vi "UserEvent Driver.vi"(0 "Message":string, 5 "Data":variant, 11 "error in (no error)":errorcluster, 13 "Operations(Get Reference)":T1=enum."Get Reference") -> (4 "user event":refnum<user-event>, 15 "error out":errorcluster)   [LabVIEW 2014, in "Coding Platform.lvlib"]
uses:
  Coding Platform.lvlib
  Typedefs/User Event Data.ctl
  Typedefs/User Event Operations.ctl
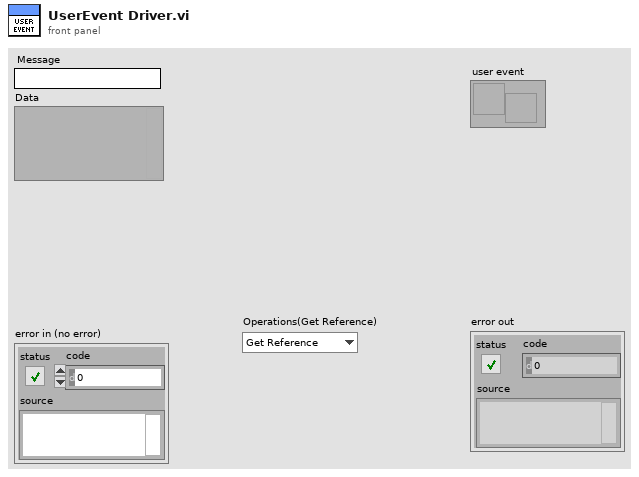
[diagram p1: front panel]
types:
  T1 = typedef "Coding Platform.lvlib/User Event Operations.ctl" = enum16{"Create", "Genereate", "Destroy", "Get Reference"}
  T2 = typedef "Coding Platform.lvlib/User Event Data.ctl" = cluster{"Message":string, "Data":variant}
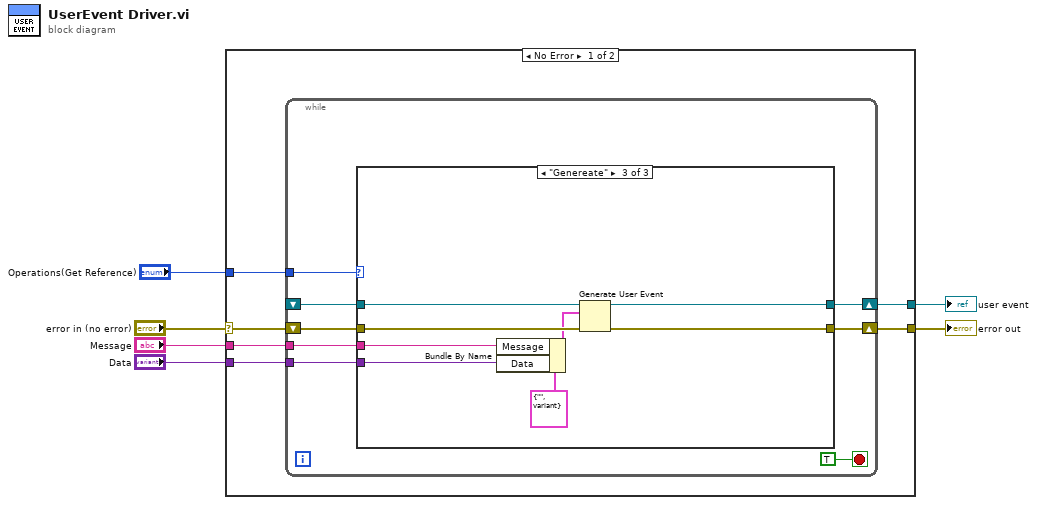
[diagram p0: block diagram]
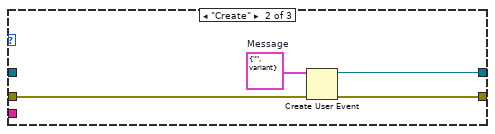
[diagram p3: hidden frame]
diagram:
  n1 = case shown="No Error" "error in (no error)" {
    selector: "error in (no error)" -> [w12 w35]
    tunnel: [w11 w35] -> w6
    tunnel: "Operations(Get Reference)" -> [w10 _]
    tunnel: [w9 _] -> w3
    tunnel: "Data" -> [w8 _]
    tunnel: "Message" -> [w7 _]
    frame No Error {
      n2 = while {
        shift-right: [w19] -> w11
        shift-left: w12 -> [w20]
        tunnel: w10 -> [w17]
        shift-right: [w16] -> w9
        shift-left: _ -> [w15]
        tunnel: w8 -> [w14]
        tunnel: w7 -> [w13]
        stop <- TRUE stop-if-true
        n3 = case shown="\"Genereate\"" w17 {
          tunnel: w20 -> [w22 w26 w34]
          tunnel: [w22 w25 w33] -> w19
          tunnel: [w21 w23 w31] -> w16
          tunnel: w15 -> [w21 _ w32]
          tunnel: w14 -> [_ _ w28]
          tunnel: w13 -> [_ _ w27]
          frame "Get Reference", Default {
          }
          frame "Create" {
            w24 = T2 {"Message"="", "Data"=variant}  # Message
            n4 = Create User Event(user event datatype=w24, error in=w26) -> (user event=w23:refnum<user-event>, error out=w25:errorcluster)
          }
          frame "Genereate" {
            n5 = Bundle By Name(cluster=T2 {"Message"="", "Data"=variant} ("event data"), "Message"=w27, "Data"=w28) -> (w29:T2)
            n6 = Generate User Event(user event=w32, event data cluster=w29, error in=w34) -> (user event out=w31:refnum<user-event>, error out=w33:errorcluster)  [unwired: 1 in]
          }
        }
      }
    }
    frame Error {
    }
  }
  "error out" <- w6
  "user event" <- w3
